vi "Datasheet Histogram Result.vi"(6 "Connection Refnum":T1, 8 "error in (no error)":errorcluster, 10 "Histogram Results":T3, 11 "Query Parameters":T5) -> (0 "error out":errorcluster, 3 "Key Array":T2)   [LabVIEW 2011]
uses:
  Datasheet Analysis Parameters.ctl
  Statistics Data.ctl
  CGI SimpleStat Results.ctl
  Addons/internet/utils/keyedarr.llb/Keyed Array.ctl
  SI.LIB/ODBC/SQL Controls/Connection Refnum.ctl
  Addons/internet/utils/strutil.llb/Case Matching.ctl
  <vilib>/Analysis/NI_AALPro.lvlib
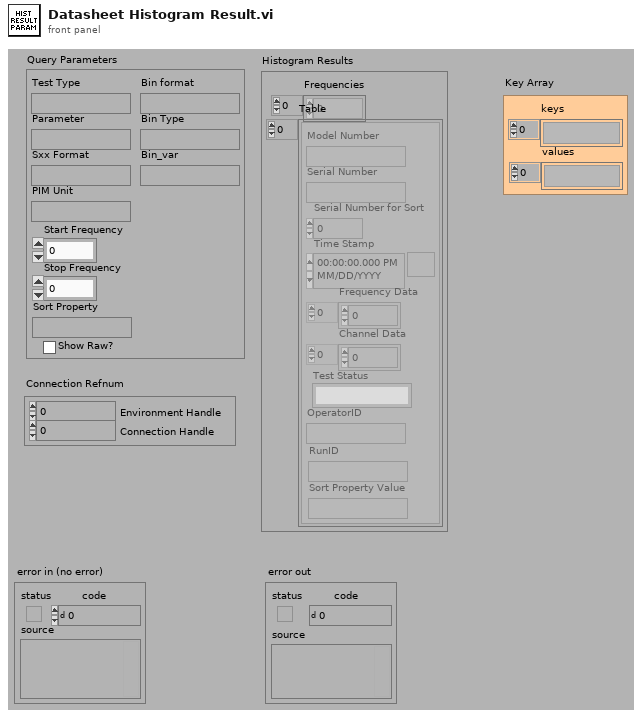
[diagram p1: front panel]
types:
  T1 = typedef "Connection Refnum.ctl" = cluster{"Environment Handle":i32, "Connection Handle":i32}
  T2 = typedef "Keyed Array.ctl" = cluster{"keys":string[], "values":string[]}
  T3 = typedef "Statistics Data.ctl" = cluster{"Table":T4[], "Frequencies":dbl[]}
  T4 = typedef "CGI SimpleStat Results.ctl" = cluster{"Model Number":string, "Serial Number for Sort":i32, "Serial Number":string, "Time Stamp":timestamp, "Channel Data":dbl[], "Test Status":string, "OperatorID":string, "Frequency Data":dbl[], "RunID":string, "Sort Property Value":string}
  T5 = typedef "Datasheet Analysis Parameters.ctl" = cluster{"Test Type":string, "Parameter":string, "Sxx Format":string, "PIM Unit":string, "Start Frequency":dbl, "Stop Frequency":dbl, "Sort Property":string, "Show Raw?":bool, "Bin format":string, "Bin Type":string, "Bin_var":string}
  T6 = typedef "Case Matching.ctl" = enum16{"a != A", "a == A", "system"}
  T7 = enum16{"Log MAG", "Lin MAG", "VSWR", "Phase", "Delay", "Insertion Loss", "Isolation", "Return Loss"}
  T8 = typedef "Field Record.ctl" = cluster{"ixField":i32, "iSequenceOrder":i32, "sxFieldId":string, "sxSequenceId":string, "sDisplayName":string, "sValue":string, "sUnits":string, "nDataType":T9, "nNextItem":T10, "fSystem":bool, "fSystemValue":bool, "fRequired":bool, "fSetAtTest":bool, "fTestField":bool, "fDeleted":bool, "fIndexed":bool, "fFreeList":bool}
  T9 = typedef "Field DataTypes.ctl" = enum32{"text", "numeric", "list", "timestamp", "boolean"}
  T10 = typedef "Field NextItem.ctl" = enum32{"Reset", "Retain", "Auto-Increment"}
  T11 = cluster{"lower":dbl, "upper":dbl, "inclusion":enum32{"lower", "upper", "both", "neither"}}[]
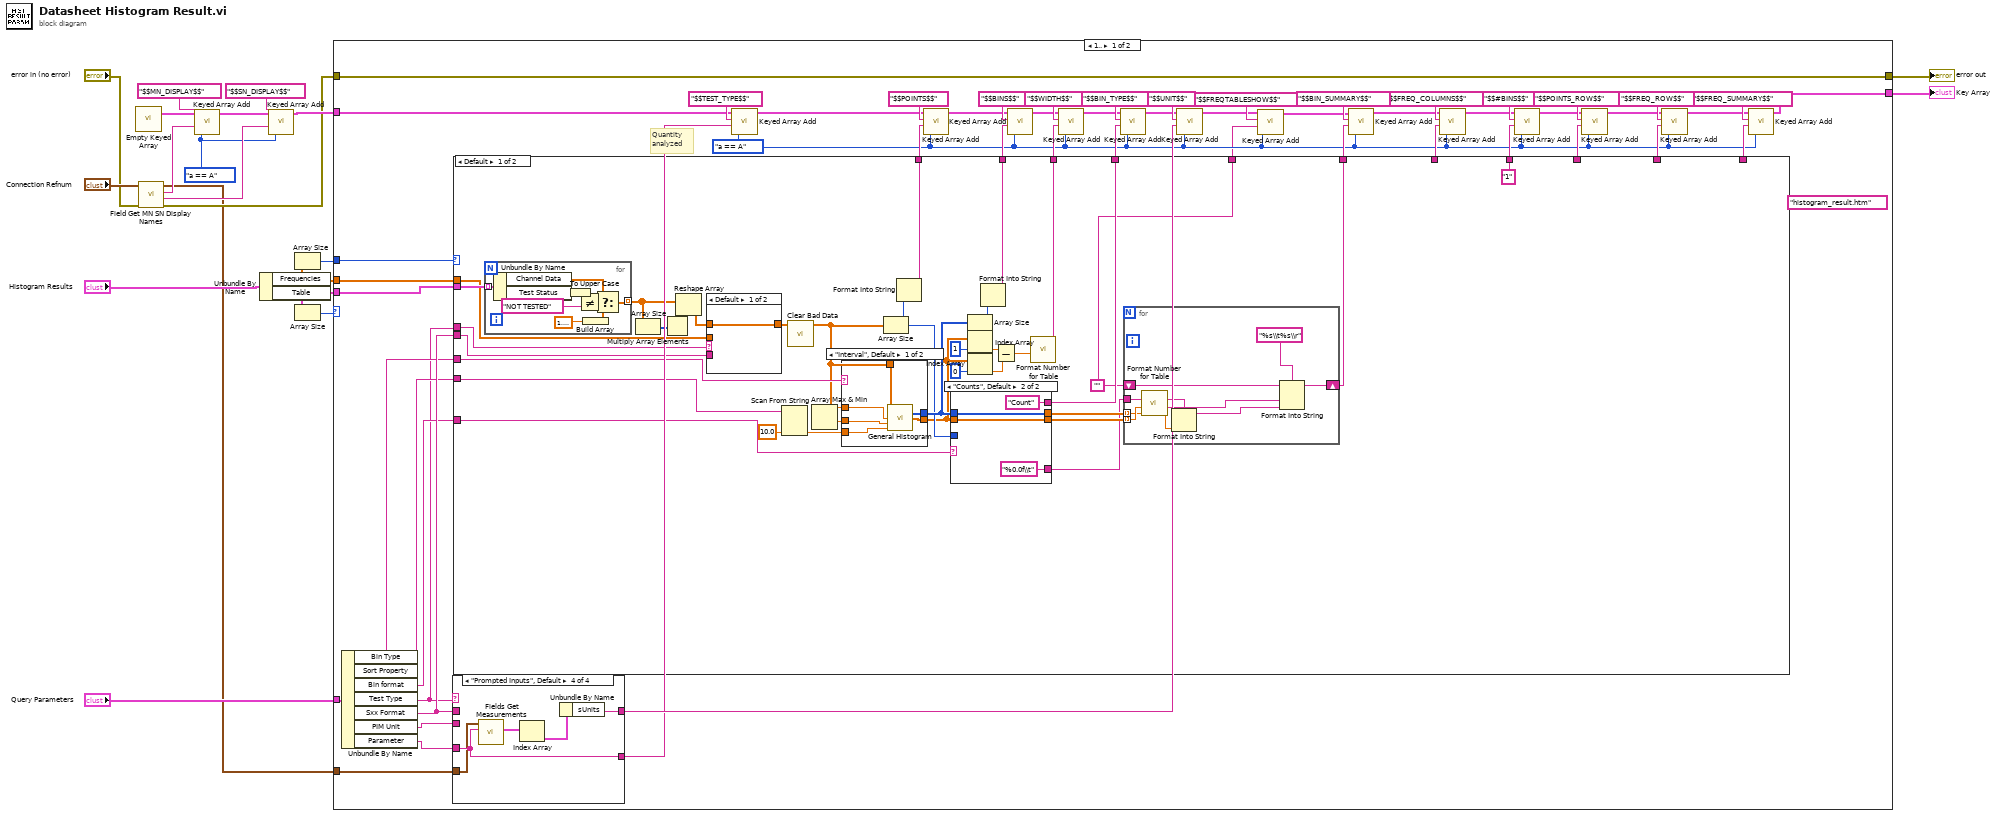
[diagram p0: block diagram]
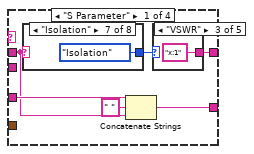
[diagram p2: hidden frame]
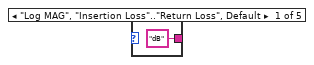
[diagram p3: hidden frame]
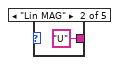
[diagram p4: hidden frame]
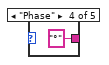
[diagram p5: hidden frame]
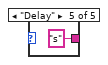
[diagram p6: hidden frame]
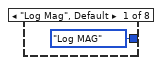
[diagram p7: hidden frame]
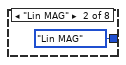
[diagram p8: hidden frame]
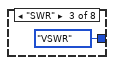
[diagram p9: hidden frame]
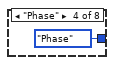
[diagram p10: hidden frame]
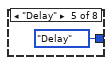
[diagram p11: hidden frame]
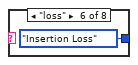
[diagram p12: hidden frame]
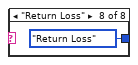
[diagram p13: hidden frame]
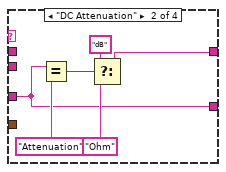
[diagram p14: hidden frame]
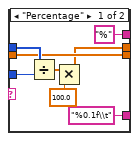
[diagram p16: hidden frame]
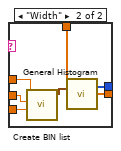
[diagram p17: hidden frame]
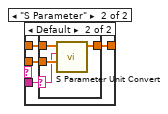
[diagram p18: hidden frame]
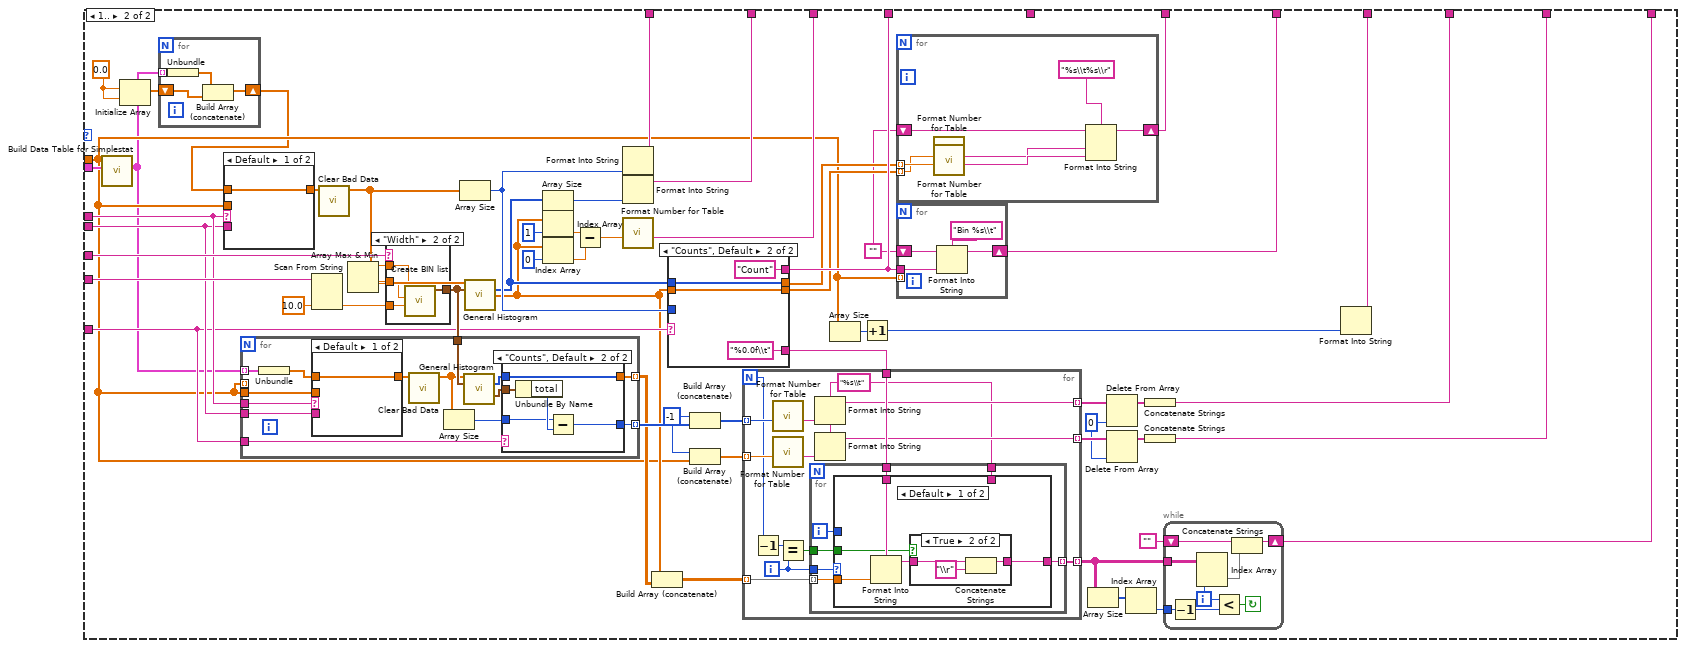
[diagram p20: hidden frame]
diagram:
  w8 = Case_Matching."a == A" ("case matching (sensitive)")
  n1 = call "Empty Keyed Array.vi"() -> ("empty keyed array"=w7:T2)  [unwired: 3 out]
  n2 = call "Field Get MN SN Display Names.vi"("error in (no error)"="error in (no error)", "Connection Refnum"="Connection Refnum") -> ("error out"=w3:errorcluster, "Serial Number Display Name"=w9:string, "Model Number Display Name"=w10:string, "Connection Refnum"=w2:T1)  [unwired: 6 out]
  n3 = call "Keyed Array Add.vi"("case matching (sensitive)"=w8, "value"=w10, "key"="$$MN_DISPLAY$$", "array in"=w7) -> ("array out"=w11:T2)  [unwired: 3 out]
  n4 = Unbundle By Name("Histogram Results") -> ("Frequencies"=w16:dbl[], "Table"=w15:T4[])
  n5 = call "Keyed Array Add.vi"("case matching (sensitive)"=w8, "value"=w9, "key"="$$SN_DISPLAY$$", "array in"=w11) -> ("array out"=w6:T2)  [unwired: 3 out]
  n6 = Array Size(array=w16) -> (size(s)=w18:i32)
  n7 = Array Size(array=w15) -> (size(s)=w14:i32)
  n8 = case shown="1.." w14 {
    tunnel: [w30 w388] -> w20
    tunnel: w3 -> [w30 w388]
    tunnel: w18 -> [w62 _]
    tunnel: "Query Parameters" -> [w61 w404]
    tunnel: w16 -> [w60 _]
    tunnel: w15 -> [w37 _]
    tunnel: w6 -> [w32 w390]
    tunnel: [w31 w389] -> w1
    tunnel: w2 -> [w21 w380]
    frame 1.. {
      (unwired) "histogram_result.htm" ("Template (\"\")")
      w27 = Case_Matching."a == A" ("case matching (sensitive)")
      # "Quantity \nanalyzed"
      n9 = Unbundle By Name(w61) -> ("Bin Type"=w58:string, "Sort Property"=w57:string, "Bin format"=w56:string, "Test Type"=w43:string, "Sxx Format"=w59:string, "PIM Unit"=w22:string, "Parameter"=w24:string)
      n10 = case shown="\"Prompted Inputs\", Default" w43 {
        tunnel: w59 -> [w76 _ _ _]
        tunnel: [w79 w95 w100 w104] -> w51
        tunnel: w24 -> [w77 w94 w101 w103]
        tunnel: [w75 w94 w101 w103] -> w23
        tunnel: w22 -> [_ _ w100 _]
        tunnel: w21 -> [_ _ _ w102]
        frame "S Parameter" {
          n11 = case shown="\"Isolation\"" w76 {
            tunnel: [T7."Log MAG" ("Display Format") T7."Lin MAG" ("Display Format") T7."VSWR" ("Display Format") T7."Phase" ("Display Format") T7."Delay" ("Display Format") T7."Insertion Loss" ("Display Format") T7."Isolation" ("Display Format") T7."Return Loss" ("Display Format")] -> w80
            frame "Log Mag", Default {
            }
            frame "Lin MAG" {
            }
            frame "SWR" {
            }
            frame "Phase" {
            }
            frame "Delay" {
            }
            frame "loss" {
            }
            frame "Isolation" {
            }
            frame "Return Loss" {
            }
          }
          n12 = Concatenate Strings(w77, " " ("search string"), w76) -> (w75:string)
          n13 = case shown="\"VSWR\"" w80 {
            tunnel: ["dB" "U" "x:1" "°" "s"] -> w79
            frame "Log MAG", "Insertion Loss".."Return Loss", Default {
            }
            frame "Lin MAG" {
            }
            frame "VSWR" {
            }
            frame "Phase" {
            }
            frame "Delay" {
            }
          }
        }
        frame "DC Attenuation" {
          n14 = Equal?(x=w94, y="Attenuation" ("search string")) -> (x = y?=w98:bool)
          n15 = Select(t="dB" ("search string"), s=w98, f="Ohm" ("search string")) -> (s? t:f=w95:string)
        }
        frame "PIM" {
        }
        frame "Prompted Inputs", Default {
          n16 = call "Fields Get Measurements.vi"("sDisplayName (empty, get all)"=w103, "Connection Refnum"=w102) -> ("Measurement Fields"=w106:T8[])  [unwired: 1 in, 8 out]
          n17 = Index Array(array=w106) -> (element=w105:T8)  [unwired: 1 in]
          n18 = Unbundle By Name(w105) -> ("sUnits"=w104:string)
        }
      }
      n19 = case shown="Default" w62 {
        tunnel: w60 -> [w137 w202]
        tunnel: w37 -> [w142 w252]
        tunnel: w43 -> [w135 w243]
        tunnel: w59 -> [w134 w242]
        tunnel: w58 -> [w133 w250]
        tunnel: w57 -> [w131 w247]
        tunnel: w56 -> [w114 w240]
        tunnel: [w120 w231] -> w55
        tunnel: [w119 w230] -> w54
        tunnel: [w118 w229] -> w53
        tunnel: [w113 w208] -> w52
        tunnel: [_ w216] -> w50
        tunnel: [_ w213] -> w47
        tunnel: [_ w219] -> w44
        tunnel: [_ w207] -> w41
        tunnel: [w109 w204] -> w39
        tunnel: ["1" w199] -> w36
        tunnel: [w107 _] -> w26
        frame Default {
          w107 = ""
          n20 = for {
            tunnel: w142 -> [w194] mode=indexing
            tunnel: [w190] -> w139 mode=indexing
            n21 = Unbundle By Name(w194) -> ("Channel Data"=w191:dbl[], "Test Status"=w193:string)
            n22 = To Upper Case(1:w193) -> (0:w186:string)
            n23 = Not Equal?(x=w186, y="NOT TESTED") -> (x != y?=w192:bool)
            n24 = Build Array(1.1447298858494002) -> (w189:dbl[])
            n25 = Select(t=w191, s=w192, f=w189) -> (s? t:f=w190:dbl[])
          }
          n26 = Array Size(array=w139) -> (size(s)=w140:i32[])
          n27 = Multiply Array Elements(1:w140) -> (0:w141:i32)
          n28 = Reshape Array(w139, w141) -> (w138:dbl[])
          n29 = case shown="Default" w135 {
            tunnel: w138 -> [w176 w180]
            tunnel: [w176 w179] -> w136
            tunnel: w134 -> [_ w177]
            tunnel: w137 -> [_ w178]
            frame Default {
            }
            frame "S Parameter" {
              n30 = case shown="Default" w177 {
                selector: w177 -> [_ w182]
                tunnel: w180 -> [w181 w185]
                tunnel: [w181 w184] -> w179
                tunnel: w178 -> [_ w183]
                frame "delay" {
                }
                frame Default {
                  n31 = call "S Parameter Unit Convert.vi"("Frequency Array"=w183, "Format"=w182, "Waveform IN"=w185) -> ("Waveform out"=w184:dbl[])  [unwired: 8 out]
                }
              }
            }
          }
          n32 = Scan From String(input string=w131, default 1=10.0 ("default value 1")) -> (output 1=w130:dbl)  [unwired: 3 in, 3 out]
          n33 = call "Clear Bad Data.vi"("Waveform IN"=w136) -> ("Waveform out"=w121:dbl[])  [unwired: 10 out]
          n34 = Array Max & Min(array=w121) -> (max value=w129:dbl, min value=w128:dbl)  [unwired: 2 out]
          n35 = case shown="\"Interval\", Default" w133 {
            tunnel: w121 -> [w166 w170]
            tunnel: [w168 w171] -> w115
            tunnel: [w167 w172] -> w117
            tunnel: w130 -> [w163 w175]
            tunnel: w129 -> [w165 w174]
            tunnel: w128 -> [w164 w173]
            frame "Interval", Default {
              n36 = call <vilib>:"General Histogram.vi"("X"=w166, "max"=w165, "min"=w164, "# bins"=w163) -> ("Histogram"=w167:i32[], "Axis"=w168:dbl[])  [unwired: 2 in, 8 out]
            }
            frame "Width" {
              n37 = call "Create BIN list.vi"("Bin Width"=w175, "Min"=w173, "Max"=w174) -> ("Bins"=w169:T11)  [unwired: 8 out]
              n38 = call <vilib>:"General Histogram.vi"("X"=w170, "Bins"=w169) -> ("Histogram"=w172:i32[], "Axis"=w171:dbl[])  [unwired: 4 in, 8 out]
            }
          }
          n39 = Array Size(array=w121) -> (size(s)=w116:i32)
          n40 = Format Into String(w116) -> (resulting string=w120:string)  [unwired: 3 in, 1 out]
          n41 = case shown="\"Counts\", Default" w114 {
            tunnel: w115 -> [w154 w162]
            tunnel: [w154 w162] -> w111
            tunnel: w117 -> [w158 w160]
            tunnel: [w152 w160] -> w112
            tunnel: w116 -> [w157 _]
            tunnel: ["%" ("search string") "Count" ("search string")] -> w113
            tunnel: ["%0.1f\\t" ("search string") "%0.0f\\t" ("search string")] -> w110
            frame "Percentage" {
              n42 = Divide(x=w158, y=w157) -> (x/y=w156:dbl[])
              n43 = Multiply(x=w156, y=100.0 ("default value 1")) -> (x*y=w152:dbl[])
            }
            frame "Counts", Default {
            }
          }
          n44 = Array Size(array=w117) -> (size(s)=w127:i32)
          n45 = Index Array(array=w115, index=1 ("disabled index (col)")) -> (element=w125:dbl)
          n46 = Index Array(array=w115, index=0 ("disabled index (col)")) -> (element=w126:dbl)
          n47 = Format Into String(w127) -> (resulting string=w119:string)  [unwired: 3 in, 1 out]
          n48 = Subtract(x=w125, y=w126) -> (x-y=w122:dbl)
          n49 = call "Format Number for Table.vi"("Number"=w122) -> ("Number String"=w118:string)  [unwired: 2 in, 8 out]
          n50 = for {
            tunnel: w111 -> [w150] mode=indexing
            tunnel: w112 -> [w145] mode=indexing
            shift-right: [w148] -> w109
            shift-left: w107 -> [w147]
            tunnel: w110 -> [w143]
            n51 = call "Format Number for Table.vi"("Number"=w150) -> ("Number String"=w146:string)  [unwired: 2 in, 8 out]
            n52 = Format Into String(format string=w143, w145) -> (resulting string=w144:string)  [unwired: 2 in, 1 out]
            n53 = Format Into String(format string="%s\\t%s\\r" ("string"), initial string=w147, w146, w144) -> (resulting string=w148:string)  [unwired: 1 in, 1 out]
          }
        }
        frame 1.. {
          w196 = 0.0 ("default value 1")
          w203 = ""
          w212 = 0 ("index")
          w226 = -1 ("disabled index (col)")
          n54 = call "Build Data Table for Simplestat.vi"("Table"=w252, "Frequency Array"=w202) -> ("All Data by Frequency"=w198:cluster{"Array":dbl[]}[])  [unwired: 9 out]
          n55 = Initialize Array(w196, w196) -> (w197:dbl[])
          n56 = for {
            tunnel: w198 -> [w256] mode=indexing
            shift-right: [w253] -> w195
            shift-left: w197 -> [w254]
            n57 = Unbundle(w256) -> ("Array"=w255:dbl[])
            n58 = Build Array (concatenate)(w255, w254) -> (w253:dbl[])
          }
          n59 = case shown="Default" w243 {
            tunnel: w195 -> [w369 w373]
            tunnel: [w369 w372] -> w251
            tunnel: w242 -> [_ w370]
            tunnel: w202 -> [_ w371]
            frame Default {
            }
            frame "S Parameter" {
              n60 = case shown="Default" w370 {
                selector: w370 -> [_ w375]
                tunnel: w373 -> [w374 w378]
                tunnel: [w374 w377] -> w372
                tunnel: w371 -> [_ w376]
                frame "delay" {
                }
                frame Default {
                  n61 = call "S Parameter Unit Convert.vi"("Frequency Array"=w376, "Format"=w375, "Waveform IN"=w378) -> ("Waveform out"=w377:dbl[])  [unwired: 8 out]
                }
              }
            }
          }
          n62 = Scan From String(input string=w247, default 1=10.0 ("default value 1")) -> (output 1=w248:dbl)  [unwired: 3 in, 3 out]
          n63 = call "Clear Bad Data.vi"("Waveform IN"=w251) -> ("Waveform out"=w241:dbl[])  [unwired: 10 out]
          n64 = Array Max & Min(array=w241) -> (max value=w246:dbl, min value=w245:dbl)  [unwired: 2 out]
          n65 = case shown="\"Width\"" w250 {
            tunnel: w248 -> [w364 w367]
            tunnel: [w363 w368] -> w244
            tunnel: w246 -> [w362 w366]
            tunnel: w245 -> [w361 w365]
            frame "Interval", Default {
              n66 = call "Create BIN list by Bin Count.vi"("Number of Bins"=w364, "Min"=w361, "Max"=w362) -> ("Bins"=w363:T11)  [unwired: 8 out]
            }
            frame "Width" {
              n67 = call "Create BIN list.vi"("Bin Width"=w367, "Min"=w365, "Max"=w366) -> ("Bins"=w368:T11)  [unwired: 8 out]
            }
          }
          n68 = for {
            tunnel: w244 -> [w337]
            tunnel: w240 -> [w335]
            tunnel: w202 -> [w328]
            tunnel: [w334] -> w224 mode=indexing
            tunnel: [w330] -> w225 mode=indexing
            tunnel: w202 -> [_] mode=indexing
            tunnel: w243 -> [w327]
            tunnel: w242 -> [w326]
            tunnel: w198 -> [w325] mode=indexing
            n69 = Unbundle(w325) -> ("Array"=w324:dbl[])
            n70 = case shown="Default" w327 {
              tunnel: w324 -> [w338 w342]
              tunnel: [w338 w341] -> w329
              tunnel: w326 -> [_ w339]
              tunnel: w328 -> [_ w340]
              frame Default {
              }
              frame "S Parameter" {
                n71 = case shown="Default" w339 {
                  selector: w339 -> [_ w344]
                  tunnel: w342 -> [w343 w347]
                  tunnel: [w343 w346] -> w341
                  tunnel: w340 -> [_ w345]
                  frame "delay" {
                  }
                  frame Default {
                    n72 = call "S Parameter Unit Convert.vi"("Frequency Array"=w345, "Format"=w344, "Waveform IN"=w347) -> ("Waveform out"=w346:dbl[])  [unwired: 8 out]
                  }
                }
              }
            }
            n73 = call "Clear Bad Data.vi"("Waveform IN"=w329) -> ("Waveform out"=w333:dbl[])  [unwired: 10 out]
            n74 = Array Size(array=w333) -> (size(s)=w331:i32)
            n75 = call <vilib>:"General Histogram.vi"("X"=w333, "Bins"=w337) -> ("Histogram"=w336:i32[], "# outside"=w332:cluster{"total":i32, "below":i32, "above":i32})  [unwired: 4 in, 8 out]
            n76 = case shown="\"Counts\", Default" w335 {
              tunnel: w336 -> [w355 w360]
              tunnel: [w352 w360] -> w334
              tunnel: w331 -> [w350 w357]
              tunnel: w332 -> [w351 w358]
              tunnel: [w348 w356] -> w330
              frame "Percentage" {
                n77 = Unbundle By Name(w351) -> ("total"=w349:i32)
                n78 = Subtract(x=w350, y=w349) -> (x-y=w348:i32)
                n79 = Divide(x=w355, y=w348) -> (x/y=w354:dbl[])
                n80 = Multiply(x=w354, y=100.0 ("default value 1")) -> (x*y=w352:dbl[])
              }
              frame "Counts", Default {
                n81 = Unbundle By Name(w358) -> ("total"=w359:i32)
                n82 = Subtract(x=w357, y=w359) -> (x-y=w356:i32)
              }
            }
          }
          n83 = Array Size(array=w241) -> (size(s)=w233:i32)
          n84 = call <vilib>:"General Histogram.vi"("X"=w241, "Bins"=w244) -> ("Histogram"=w232:i32[], "Axis"=w223:dbl[])  [unwired: 4 in, 8 out]
          n85 = Array Size(array=w232) -> (size(s)=w239:i32)
          n86 = Index Array(array=w223, index=1 ("disabled index (col)")) -> (element=w237:dbl)
          n87 = Index Array(array=w223, index=0 ("disabled index (col)")) -> (element=w238:dbl)
          n88 = Subtract(x=w237, y=w238) -> (x-y=w234:dbl)
          n89 = Format Into String(w233) -> (resulting string=w231:string)  [unwired: 3 in, 1 out]
          n90 = Format Into String(w239) -> (resulting string=w230:string)  [unwired: 3 in, 1 out]
          n91 = call "Format Number for Table.vi"("Number"=w234) -> ("Number String"=w229:string)  [unwired: 2 in, 8 out]
          n92 = Build Array (concatenate)(w223, w224) -> (w221:dbl[][])
          n93 = case shown="\"Counts\", Default" w240 {
            tunnel: w223 -> [w315 w323]
            tunnel: [w315 w323] -> w205
            tunnel: w232 -> [w319 w321]
            tunnel: [w313 w321] -> w206
            tunnel: w233 -> [w318 _]
            tunnel: ["Percentage" ("search string") "Count" ("search string")] -> w208
            tunnel: ["%0.1f\\t" ("search string") "%0.0f\\t" ("search string")] -> w222
            frame "Percentage" {
              n94 = Divide(x=w319, y=w318) -> (x/y=w317:dbl[])
              n95 = Multiply(x=w317, y=100.0 ("default value 1")) -> (x*y=w313:dbl[])
            }
            frame "Counts", Default {
            }
          }
          n96 = Build Array (concatenate)(w226, w225) -> (w227:i32[])
          n97 = Build Array (concatenate)(w226, w202) -> (w228:dbl[])
          n98 = for {
            N -> [w283]
            tunnel: w221 -> [w289] mode=indexing
            tunnel: w222 -> [w288]
            tunnel: w227 -> [w286] mode=indexing
            tunnel: w228 -> [w287] mode=indexing
            tunnel: [w279] -> w211 mode=indexing
            tunnel: [w278] -> w218 mode=indexing
            tunnel: [w277] -> w214 mode=indexing
            i -> [w281]
            w276 = "%s\\t" ("format string")
            n99 = Decrement(x=w283) -> (x-1=w282:i32)
            n100 = call "Format Number for Table.vi"("Number"=w286) -> ("Number String"=w285:string)  [unwired: 2 in, 8 out]
            n101 = call "Format Number for Table.vi"("Number"=w287) -> ("Number String"=w284:string)  [unwired: 2 in, 8 out]
            n102 = Equal?(x=w282, y=w281) -> (x = y?=w280:bool)
            n103 = for {
              tunnel: w289 -> [w295] mode=indexing
              tunnel: w288 -> [w294]
              tunnel: w281 -> [w293]
              tunnel: w280 -> [w291]
              tunnel: [w296] -> w279 mode=indexing
              tunnel: w276 -> [w290]
              i -> [w292]
              n104 = case shown="Default" w293 {
                tunnel: [w297 w309] -> w296
                tunnel: w295 -> [w301 w311]
                tunnel: w294 -> [w300 _]
                tunnel: w292 -> [_ _]
                tunnel: w291 -> [w299 _]
                tunnel: w290 -> [_ w307]
                frame Default {
                  n105 = Format Into String(format string=w300, w301) -> (resulting string=w298:string)  [unwired: 2 in, 1 out]
                  n106 = case shown="True" w299 {
                    tunnel: w298 -> [w302 w305]
                    tunnel: [w302 w304] -> w297
                    frame False {
                    }
                    frame True {
                      n107 = Concatenate Strings(w305, "\\r" ("string")) -> (w304:string)
                    }
                  }
                }
                frame 0 {
                  n108 = call "Format Number for Table.vi"("Number"=w311) -> ("Number String"=w310:string)  [unwired: 3 in, 7 out]
                  n109 = Concatenate Strings("\\r", w307) -> (w308:string)
                  n110 = Format Into String(format string=w308, w310) -> (resulting string=w309:string)  [unwired: 2 in, 1 out]
                }
              }
            }
            n111 = Format Into String(format string=w276, w285) -> (resulting string=w278:string)  [unwired: 2 in, 1 out]
            n112 = Format Into String(format string=w276, w284) -> (resulting string=w277:string)  [unwired: 2 in, 1 out]
          }
          n113 = Array Size(array=w202) -> (size(s)=w201:i32)
          n114 = Increment(x=w201) -> (x+1=w200:i32)
          n115 = for {
            tunnel: w205 -> [w262] mode=indexing
            tunnel: w206 -> [w263] mode=indexing
            shift-right: [w260] -> w204
            shift-left: w203 -> [w259]
            n116 = call "Format Number for Table.vi"("Number"=w262) -> ("Number String"=w257:string)  [unwired: 2 in, 8 out]
            n117 = call "Format Number for Table.vi"("Number"=w263) -> ("Number String"=w258:string)  [unwired: 2 in, 8 out]
            n118 = Format Into String(format string="%s\\t%s\\r" ("string"), initial string=w259, w257, w258) -> (resulting string=w260:string)  [unwired: 1 in, 1 out]
          }
          n119 = for {
            tunnel: w202 -> [_] mode=indexing
            shift-right: [w266] -> w207
            shift-left: w203 -> [w265]
            tunnel: w208 -> [w264]
            n120 = Format Into String(format string="Bin %s\\t" ("string"), initial string=w265, w264) -> (resulting string=w266:string)  [unwired: 1 in, 1 out]
          }
          n121 = Array Size(array=w211) -> (size(s)=w210:i32[])
          n122 = Delete From Array(array=w218, index=w212) -> (array with subset deleted=w217:string[])  [unwired: 1 in, 1 out]
          n123 = Delete From Array(array=w214, index=w212) -> (array with subset deleted=w215:string[])  [unwired: 1 in, 1 out]
          n124 = Index Array(array=w210) -> (element=w209:i32)  [unwired: 1 in]
          n125 = Concatenate Strings(w217) -> (w216:string)
          n126 = Concatenate Strings(w215) -> (w213:string)
          n127 = while {
            tunnel: w211 -> [w270]
            shift-right: [w275] -> w219
            shift-left: "" -> [w274]
            tunnel: w209 -> [w272]
            i -> [w268]
            stop <- w271 continue-if-true
            n128 = Decrement(x=w272) -> (x-1=w273:i32)
            n129 = Index Array(array=w270, index (col)=w268) -> (element=w269:string[])  [unwired: 1 in]
            n130 = Less?(x=w268, y=w273) -> (x < y?=w271:bool)
            n131 = Concatenate Strings(w274, w269) -> (w275:string)
          }
          n132 = Format Into String(w200) -> (resulting string=w199:string)  [unwired: 3 in, 1 out]
        }
      }
      n133 = call "Keyed Array Add.vi"("case matching (sensitive)"=w27, "value"=w23, "key"="$$TEST_TYPE$$", "array in"=w32) -> ("array out"=w67:T2)  [unwired: 3 out]
      n134 = call "Keyed Array Add.vi"("case matching (sensitive)"=w27, "value"=w55, "key"="$$POINTS$$", "array in"=w67) -> ("array out"=w66:T2)  [unwired: 3 out]
      n135 = call "Keyed Array Add.vi"("case matching (sensitive)"=w27, "value"=w54, "key"="$$BINS$$", "array in"=w66) -> ("array out"=w65:T2)  [unwired: 3 out]
      n136 = call "Keyed Array Add.vi"("case matching (sensitive)"=w27, "value"=w53, "key"="$$WIDTH$$", "array in"=w65) -> ("array out"=w64:T2)  [unwired: 3 out]
      n137 = call "Keyed Array Add.vi"("case matching (sensitive)"=w27, "value"=w52, "key"="$$BIN_TYPE$$", "array in"=w64) -> ("array out"=w63:T2)  [unwired: 3 out]
      n138 = call "Keyed Array Add.vi"("case matching (sensitive)"=w27, "value"=w51, "key"="$$UNIT$$", "array in"=w63) -> ("array out"=w28:T2)  [unwired: 3 out]
      n139 = call "Keyed Array Add.vi"("case matching (sensitive)"=w27, "value"=w26, "key"="$$FREQTABLESHOW$$", "array in"=w28) -> ("array out"=w25:T2)  [unwired: 3 out]
      n140 = call "Keyed Array Add.vi"("case matching (sensitive)"=w27, "value"=w39, "key"="$$BIN_SUMMARY$$", "array in"=w25) -> ("array out"=w38:T2)  [unwired: 3 out]
      n141 = call "Keyed Array Add.vi"("case matching (sensitive)"=w27, "value"=w41, "key"="$$FREQ_COLUMNS$$", "array in"=w38) -> ("array out"=w34:T2)  [unwired: 3 out]
      n142 = call "Keyed Array Add.vi"("case matching (sensitive)"=w27, "value"=w36, "key"="$$#BINS$$", "array in"=w34) -> ("array out"=w33:T2)  [unwired: 3 out]
      n143 = call "Keyed Array Add.vi"("case matching (sensitive)"=w27, "value"=w50, "key"="$$POINTS_ROW$$", "array in"=w33) -> ("array out"=w48:T2)  [unwired: 3 out]
      n144 = call "Keyed Array Add.vi"("case matching (sensitive)"=w27, "value"=w47, "key"="$$FREQ_ROW$$", "array in"=w48) -> ("array out"=w45:T2)  [unwired: 3 out]
      n145 = call "Keyed Array Add.vi"("case matching (sensitive)"=w27, "value"=w44, "key"="$$FREQ_SUMMARY$$", "array in"=w45) -> ("array out"=w31:T2)  [unwired: 3 out]
    }
    frame 0, Default {
      w379 = ""
      w385 = Case_Matching."a == A" ("case matching (sensitive)")
      # "Quantity \nanalyzed"
      n146 = Unbundle By Name(w404) -> ("Test Type"=w397:string, "Sxx Format"=w403:string, "PIM Unit"=w381:string, "Parameter"=w383:string)  [unwired: 3 out]
      n147 = case shown="\"Prompted Inputs\", Default" w397 {
        tunnel: w403 -> [w418 _ _ _]
        tunnel: [w421 w437 w442 w446] -> w402
        tunnel: w383 -> [w419 w436 w443 w445]
        tunnel: [w417 w436 w443 w445] -> w382
        tunnel: w381 -> [_ _ w442 _]
        tunnel: w380 -> [_ _ _ w444]
        frame "S Parameter" {
          n148 = case shown="\"Isolation\"" w418 {
            tunnel: [T7."Log MAG" ("Display Format") T7."Lin MAG" ("Display Format") T7."VSWR" ("Display Format") T7."Phase" ("Display Format") T7."Delay" ("Display Format") T7."Insertion Loss" ("Display Format") T7."Isolation" ("Display Format") T7."Return Loss" ("Display Format")] -> w422
            frame "Log Mag", Default {
            }
            frame "Lin MAG" {
            }
            frame "SWR" {
            }
            frame "Phase" {
            }
            frame "Delay" {
            }
            frame "loss" {
            }
            frame "Isolation" {
            }
            frame "Return Loss" {
            }
          }
          n149 = Concatenate Strings(w419, " " ("search string"), w418) -> (w417:string)
          n150 = case shown="\"VSWR\"" w422 {
            tunnel: ["dB" "U" "x:1" "°" "s"] -> w421
            frame "Log MAG", "Insertion Loss".."Return Loss", Default {
            }
            frame "Lin MAG" {
            }
            frame "VSWR" {
            }
            frame "Phase" {
            }
            frame "Delay" {
            }
          }
        }
        frame "DC Attenuation" {
          n151 = Equal?(x=w436, y="Attenuation" ("search string")) -> (x = y?=w440:bool)
          n152 = Select(t="dB" ("search string"), s=w440, f="Ohm" ("search string")) -> (s? t:f=w437:string)
        }
        frame "PIM" {
        }
        frame "Prompted Inputs", Default {
          n153 = call "Fields Get Measurements.vi"("sDisplayName (empty, get all)"=w445, "Connection Refnum"=w444) -> ("Measurement Fields"=w448:T8[])  [unwired: 1 in, 8 out]
          n154 = Index Array(array=w448) -> (element=w447:T8)  [unwired: 1 in]
          n155 = Unbundle By Name(w447) -> ("sUnits"=w446:string)
        }
      }
      n156 = call "Keyed Array Add.vi"("case matching (sensitive)"=w385, "value"=w382, "key"="$$TEST_TYPE$$", "array in"=w390) -> ("array out"=w409:T2)  [unwired: 3 out]
      n157 = call "Keyed Array Add.vi"("case matching (sensitive)"=w385, "value"=w379, "key"="$$POINTS$$", "array in"=w409) -> ("array out"=w408:T2)  [unwired: 3 out]
      n158 = call "Keyed Array Add.vi"("case matching (sensitive)"=w385, "value"=w379, "key"="$$BINS$$", "array in"=w408) -> ("array out"=w407:T2)  [unwired: 3 out]
      n159 = call "Keyed Array Add.vi"("case matching (sensitive)"=w385, "value"=w379, "key"="$$WIDTH$$", "array in"=w407) -> ("array out"=w406:T2)  [unwired: 3 out]
      n160 = call "Keyed Array Add.vi"("case matching (sensitive)"=w385, "value"=w379, "key"="$$BIN_TYPE$$", "array in"=w406) -> ("array out"=w405:T2)  [unwired: 3 out]
      n161 = call "Keyed Array Add.vi"("case matching (sensitive)"=w385, "value"=w402, "key"="$$UNIT$$", "array in"=w405) -> ("array out"=w386:T2)  [unwired: 3 out]
      n162 = call "Keyed Array Add.vi"("case matching (sensitive)"=w385, "value"=w379, "key"="$$FREQTABLESHOW$$", "array in"=w386) -> ("array out"=w384:T2)  [unwired: 3 out]
      n163 = call "Keyed Array Add.vi"("case matching (sensitive)"=w385, "value"=w379, "key"="$$BIN_SUMMARY$$", "array in"=w384) -> ("array out"=w394:T2)  [unwired: 3 out]
      n164 = call "Keyed Array Add.vi"("case matching (sensitive)"=w385, "value"=w379, "key"="$$FREQ_COLUMNS$$", "array in"=w394) -> ("array out"=w392:T2)  [unwired: 3 out]
      n165 = call "Keyed Array Add.vi"("case matching (sensitive)"=w385, "value"=w379, "key"="$$#BINS$$", "array in"=w392) -> ("array out"=w391:T2)  [unwired: 3 out]
      n166 = call "Keyed Array Add.vi"("case matching (sensitive)"=w385, "value"=w379, "key"="$$POINTS_ROW$$", "array in"=w391) -> ("array out"=w400:T2)  [unwired: 3 out]
      n167 = call "Keyed Array Add.vi"("case matching (sensitive)"=w385, "value"=w379, "key"="$$FREQ_ROW$$", "array in"=w400) -> ("array out"=w398:T2)  [unwired: 3 out]
      n168 = call "Keyed Array Add.vi"("case matching (sensitive)"=w385, "value"=w379, "key"="$$FREQ_SUMMARY$$", "array in"=w398) -> ("array out"=w389:T2)  [unwired: 3 out]
    }
  }
  "error out" <- w20
  "Key Array" <- w1
